vi "Addon.Version.Upgrade.vi"(8 "error in (no error)":errorcluster, 11 "Device Item Ref in in":T1 format="%.0x") -> (0 "error out":errorcluster, 3 "Device Item Ref out":T1 format="%.0x")   [LabVIEW 2019, in "Diagnostics Addon System Explorer.lvlib"]
uses:
  Diagnostics Addon System Explorer.lvlib
  Shared/Types/Type.ctl
  Shared/Diagnostics Addon Shared.lvlib
  <vilib>/NI VeriStand/Custom Device Tools/Custom Device Utility Library/Custom Device Utility Library.lvlib
  <vilib>/NI VeriStand/Custom Device Tools/Custom Device Utility Library/NI VeriStand - Search for Item by GUID.vi
  Types/FG.Action.ctl
  <vilib>/NI VeriStand/Custom Device API/Custom Device Channel Type.ctl
  <vilib>/NI VeriStand/Custom Device API/Custom Device API.lvlib
  <vilib>/NI VeriStand/Custom Device API/Custom Device Channel.ctl
  Types/Settings.Channel.ctl
  Shared/SubVIs/Constants.vi
  <vilib>/NI VeriStand/Custom Device API/Get Item Property (String).vi
  NationalInstruments.VeriStand.SystemDefinitionAPI
  <vilib>/NI VeriStand/Custom Device API/Custom Device Item Ref.ctl
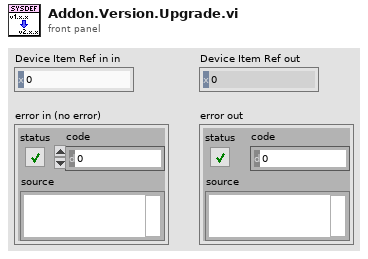
[diagram p1: front panel]
types:
  T1 = typedef "Custom Device API.lvlib/Custom Device Item Ref.ctl" = u64
  T2 = typedef "Diagnostics Addon Shared.lvlib/Type.ctl" = enum16{"DID", "CDID", "PID", "CPID", "Read Memory", "Write Memory", "IO Control", "Routine Start", "Routine Request", "Routine Stop", "User Defined", "DTC Control", "Clear DTCs", "Read DTCs", "Start DTCs", "DTC Change Count", "Tester Present", "Unlock ECU", "Reset ECU", "Diag Session Control", "Communication Control", "DPID Control", "Poll Control", "Diag CAN Control"}
  T3 = typedef "Diagnostics Addon System Explorer.lvlib/FG.Action.ctl" = enum16{"Get", "Set"}
  T4 = typedef "Diagnostics Addon Shared.lvlib/Security.ctl" = cluster{"Type":T5, "Source DLL Path":path, "Target DLL Path":path, "Security Level":u8}
  T5 = typedef "Diagnostics Addon Shared.lvlib/Security.Type.ctl" = enum16{"None", "DLL", "MasterKey"}
  T6 = typedef "Diagnostics Addon System Explorer.lvlib/Settings.Channel.ctl" = cluster{"Name":string, "Description":string, "Channel":T7}
  T7 = typedef "Custom Device API.lvlib/Custom Device Channel.ctl" = cluster{"Type":T8, "Units":string, "Default Value":dbl, "Faultable":bool, "Scalable":bool}
  T8 = typedef "Custom Device API.lvlib/Custom Device Channel Type.ctl" = enum16{"Input", "Output"}
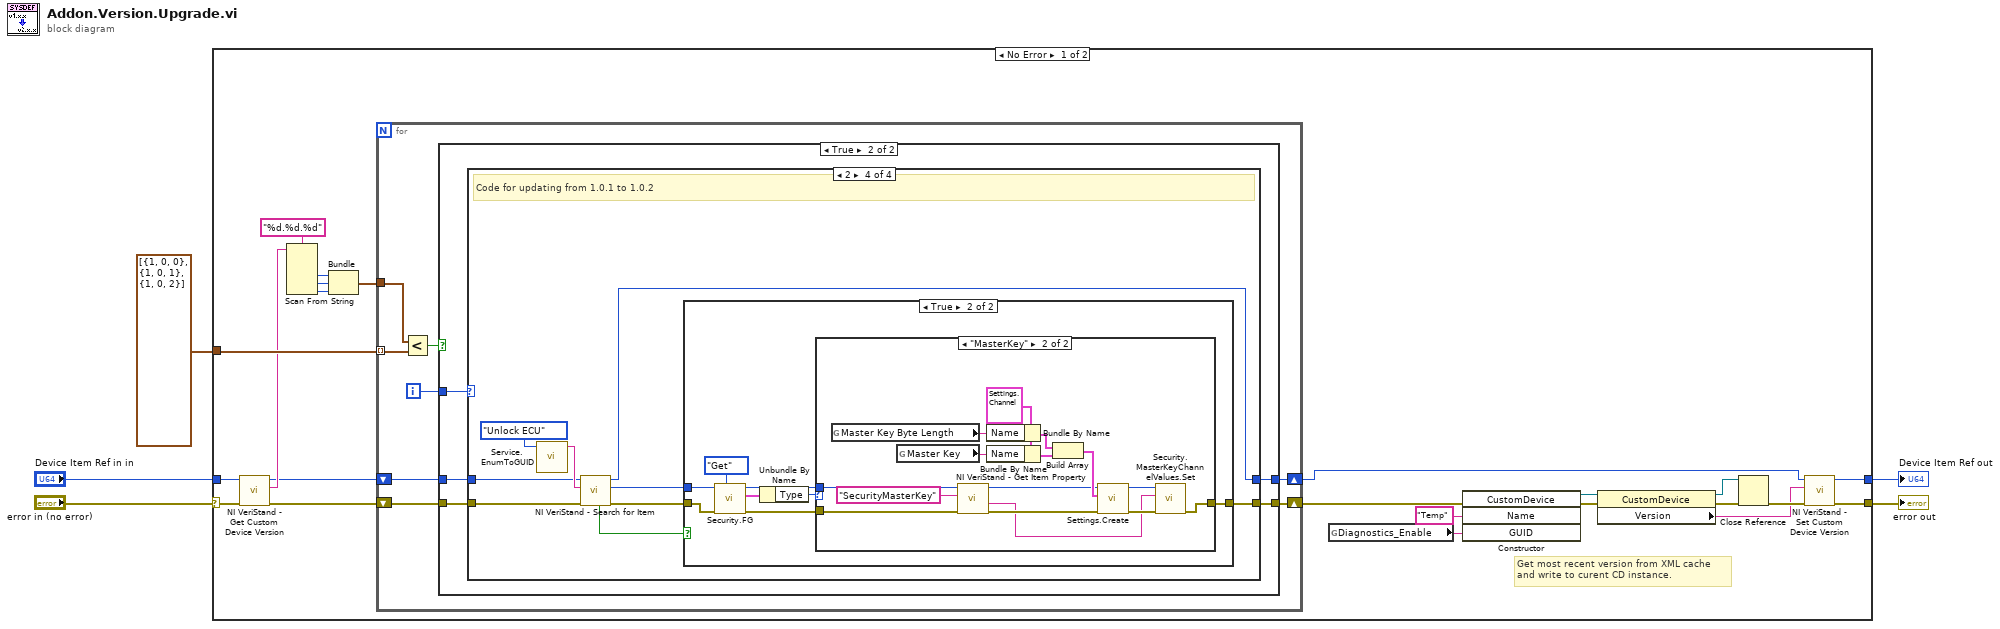
[diagram p0: block diagram]
diagram:
  n1 = case shown="No Error" "error in (no error)" {
    selector: "error in (no error)" -> [w11 w85]
    tunnel: [w21 w85] -> w4
    tunnel: "Device Item Ref in in" -> [w10 w84]
    tunnel: [w20 w84] -> w5
    tunnel: cluster{i32, i32, i32}[] [{1, 0, 0}, {1, 0, 1}, {1, 0, 2}] -> [w28 _]
    frame No Error {
      # "Get most recent version from XML cache\nand write to curent CD instance."
      n2 = call <vilib>:"NI VeriStand - Get Custom Device Version.vi"("error in (no error)"=w11, "Device Ref in"=w10) -> ("error out"=w7:errorcluster, "Value"=w15:string, "Device Ref out"=w6:T1)  [unwired: 7 in]
      n3 = Scan From String(format string="%d.%d.%d", input string=w15) -> (output 1=w13:i32, output 2=w12:i32, output 3=w14:i32)  [unwired: 5 in, 3 out]
      n4 = Bundle(w13, w12, w14) -> (w8:cluster{i32, i32, i32})  [unwired: 1 in]
      n5 = for {
        tunnel: w28 -> [w34] mode=indexing
        shift-right: [w36] -> w19
        shift-left: w7 -> [w30]
        shift-right: [w35] -> w18
        shift-left: w6 -> [w29]
        tunnel: w8 -> [w31]
        i -> [w32]
        n6 = Less?(x=w31, y=w34) -> (x < y?=w33:bool)
        n7 = case shown="True" w33 {
          tunnel: w30 -> [w38 w43]
          tunnel: [w38 w42] -> w36
          tunnel: w29 -> [w37 w39]
          tunnel: [w37 w40] -> w35
          tunnel: w32 -> [_ w41]
          frame False {
          }
          frame True {
            n8 = case shown="2" w41 {
              tunnel: w43 -> [w45 w47 w49 w56]
              tunnel: [w45 w47 w49 w50] -> w42
              tunnel: [w44 w46 w48 w55] -> w40
              tunnel: w39 -> [w44 w46 w48 w54]
              frame Default {
                # "Nothing to update"
              }
              frame 0 {
                # "Initial Onload"
              }
              frame 1 {
                # "Code for updating from 1.0.0 to 1.0.1"
              }
              frame 2 {
                # "Code for updating from 1.0.1 to 1.0.2"
                n9 = call "Service.EnumToGUID.vi"("Type"=Type."Unlock ECU") -> ("GUID"=w57:string)  [unwired: 10 in]
                n10 = call-poly <vilib>:"NI VeriStand - Search for Item.vi"("error in"=w56, "Item GUID"=w57, "Section Ref in"=w54) -> ("error out"=w52:errorcluster, "Item Ref"=w51:T1, "Section Ref out"=w55:T1, "Found"=w53:bool)  [unwired: 5 in]
                n11 = case shown="True" w53 {
                  tunnel: w52 -> [w59 w67]
                  tunnel: w51 -> [_ w66]
                  tunnel: [w59 w60] -> w50
                  frame False {
                  }
                  frame True {
                    n12 = call "Security.FG.vi"("Action"=FG.Action."Get", "error in (no error)"=w67, "Device Item Ref in"=w66) -> ("error out"=w62:errorcluster, "Security"=w64:T4, "Device Item Ref out"=w61:T1)  [unwired: 6 in]
                    n13 = Unbundle By Name(w64) -> ("Type"=w63:T5)
                    n14 = case shown="\"MasterKey\"" w63 {
                      tunnel: w62 -> [w68 w75]
                      tunnel: w61 -> [_ w73]
                      tunnel: [w68 w69] -> w60
                      frame Default {
                      }
                      frame "MasterKey" {
                        w78 = T6 {"Name"="Byte Length", "Description"="", "Channel"={"Type"=enum."Input", "Units"="", "Default Value"=0.0, "Faultable"=FALSE, "Scalable"=FALSE}} ("cluster")
                        n15 = global read "Constants.vi" "Master Key Byte Length"() -> (w80:string)
                        n16 = global read "Constants.vi" "Master Key"() -> (w79:string)
                        n17 = call-poly <vilib>:"NI VeriStand - Get Item Property.vi"("error in (no error)"=w75, "Property Name"="SecurityMasterKey" ("CAN.SecurityMasterKey"), "Item Ref in"=w73) -> ("error out"=w76:errorcluster, "Value"=w70:string, "Item Ref out"=w74:T1)  [unwired: 5 in, 1 out]
                        n18 = Bundle By Name(cluster=w78, "Name"=w80) -> (w81:T6)
                        n19 = Bundle By Name(cluster=w78, "Name"=w79) -> (w83:T6)
                        n20 = Build Array(w81, w83) -> (w82:T6[])
                        n21 = call "Settings.Create.vi"("error in (no error)"=w76, "Settings Channels"=w82, "Section Ref in"=w74) -> ("error out"=w72:errorcluster, "nodeID out"=w71:u64)  [unwired: 7 in]
                        n22 = call "Security.MasterKeyChannelValues.Set.vi"("error in (no error)"=w72, "Master Key"=w70, "Device Item Ref in"=w71) -> ("error out"=w69:errorcluster)  [unwired: 7 in, 1 out]
                      }
                    }
                  }
                }
              }
            }
          }
        }
      }
      n23 = global read "Constants.vi" "Diagnostics_Enable"() -> (w16:string)
      n24 = constructor class="CustomDevice"(error in=w19, "Name"="Temp", "GUID"=w16) -> (reference out=w27:refnum<k24>, error out=w26:errorcluster)  [unwired: 2 in, 3 out]
      n25 = property class="CustomDevice"(reference=w27, error in=w26) -> (reference out=w24:refnum<k24>, error out=w25:errorcluster, "Version"=w22:string)
      n26 = Close Reference(reference=w24, error in (no error)=w25) -> (error out=w23:errorcluster)
      n27 = call <vilib>:"NI VeriStand - Set Custom Device Version.vi"("error in (no error)"=w23, "Value"=w22, "Device Ref in"=w18) -> ("error out"=w21:errorcluster, "Device Ref out"=w20:T1)  [unwired: 7 in]
    }
    frame Error {
    }
  }
  "Device Item Ref out" <- w5
  "error out" <- w4
